vi "New.vi"(8 "error in (no error)":errorcluster) -> (0 "error out":errorcluster, 3 "Timer out":refnum<class "Timer.lvclass">)   [LabVIEW 2020, in "Timer.lvclass"]
uses:
  Timer.lvclass
  Timer.lvclass/Timer.ctl
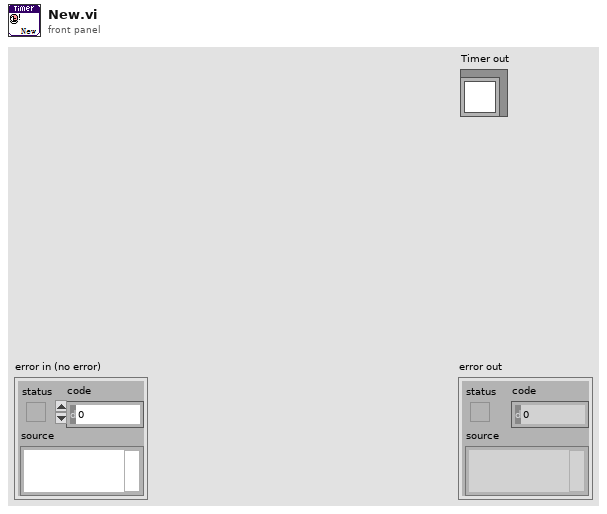
[diagram p1: front panel]
types:
  T1 = cluster{"target time(ms)":u32, "elapsed time(ms)":u32, "start time":u32, "pause":bool, "auto reset":bool}
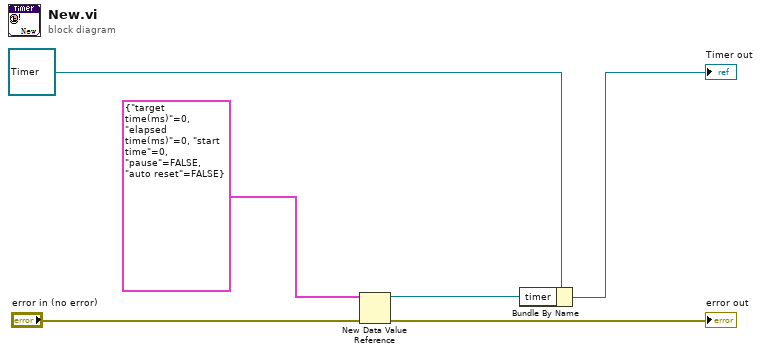
[diagram p0: block diagram]
diagram:
  n1 = New Data Value Reference(data value=T1 {"target time(ms)"=0, "elapsed time(ms)"=0, "start time"=0, "pause"=FALSE, "auto reset"=FALSE} ("output cluster"), error in="error in (no error)") -> (data value reference=w1:refnum<data-value>, error out=→"error out":errorcluster)
  n2 = Bundle By Name(cluster=refnum<class "Timer.lvclass"> refnum ("Timer in"), "timer"=w1) -> (→"Timer out":refnum<class "Timer.lvclass">)
